vi "boolandNum.vi"() -> ()   [LabVIEW 2021]
uses:
  <vilib>/numeric/Random Number (Range) I64.vi
  <vilib>/numeric/sub_Random U32.vi
panel:
  out "rand":dbl
  out "sq":dbl
  out "root":dbl
  in  "Boolean 4":bool
  in  "Boolean 3":bool
  in  "Boolean 2":bool
  out "div":dbl
  out "mult":dbl
  out "sub":dbl
  out "add":dbl
  in  "num2":dbl
  in  "num1":dbl
  out "light":bool
  in  "Boolean":bool
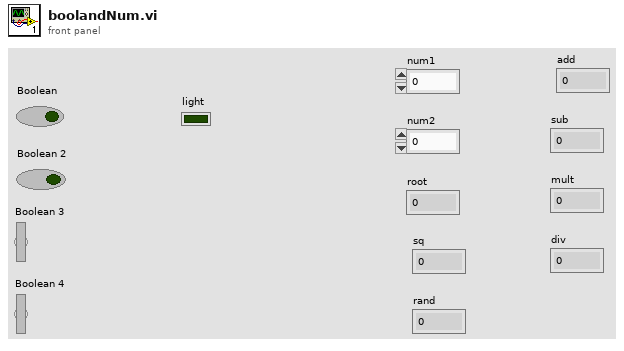
[diagram p1: front panel]
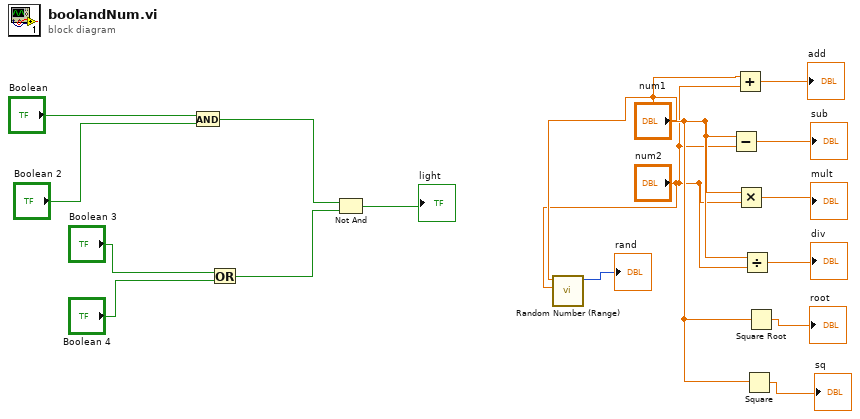
[diagram p0: block diagram]
diagram:
  n1 = And(x="Boolean", y="Boolean 2") -> (x .and. y?=w8:bool)
  n2 = Or(x="Boolean 3", y="Boolean 4") -> (x .or. y?=w7:bool)
  n3 = Not And(1:w7, 2:w8) -> (0:→"light":bool)
  n4 = call-poly <vilib>:"Random Number (Range).vi"("lower bound (-100)"="num2", "upper bound (100)"="num1") -> ("number"=→"rand":i64)  [unwired: 9 in]
  n5 = Subtract(x="num1", y="num2") -> (x-y=→"sub":dbl)
  n6 = Add(x="num1", y="num2") -> (x+y=→"add":dbl)
  n7 = Multiply(x="num1", y="num2") -> (x*y=→"mult":dbl)
  n8 = Divide(x="num1", y="num2") -> (x/y=→"div":dbl)
  n9 = Square(x="num1") -> (x^2=→"sq":dbl)
  n10 = Square Root(x="num1") -> (sqrt(x)=→"root":dbl)
